vi "LurchTowardsPoint.vi"(2 "Turning Radius (m) \n(Goes into Dillons' Movement Control)":dbl=1.75, 3 "Robot Speed":dbl(slide)=1.0 scale=0.0..1.0, 4 "Reached Next Path Point Threshold Distance (m)":dbl(knob)=0.4965904536247452 scale=0.0..1.0, 5 "Dest. Point":cluster{"x":dbl, "y":dbl}, 7 "Curr Localization Status":T1) -> (0 "Within Tolerance of Dest":bool, 1 "Distance to Dest Point (m)":dbl)   [LabVIEW 2015, in "Navigation2017.lvlib"]
doc: "Tries to move the robot one \"jump\" forward towards (or even to) a given point. Uses a time measured in the testing arena to determine a minimum time to move robot forward, erring on the side of undershooting the target point on BP-1. Likely will not exactly reach the final point, as dead reckoning is used to move bot until it stops and checks its location again."
uses:
  Navigation2017.lvlib
  LocalizationStatus.ctl
  Navigation2017-util.lvlib
  MovementControl2017.lvlib
  Navigation2017-SubVIs.lvlib
panel:
  in  "Time to move 1m (TODO: consider speed?)":u32=1
  # "INTERNAL VALUE\nTO VI:"
  # "INPUTS"
  # "OUTPUTS:"
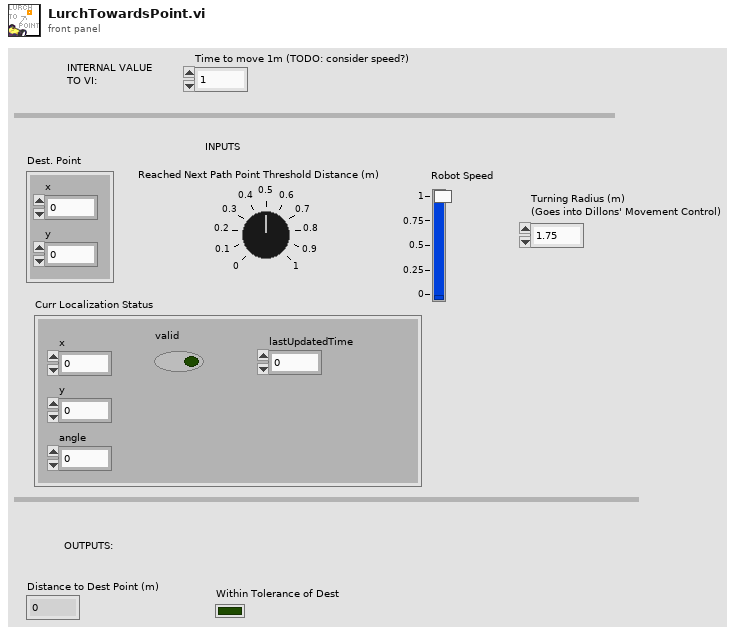
[diagram p1: front panel]
types:
  T1 = typedef "LocalizationStatus.ctl" = cluster{"x":dbl, "y":dbl, "angle":dbl, "valid":bool, "lastUpdatedTime":dbl}
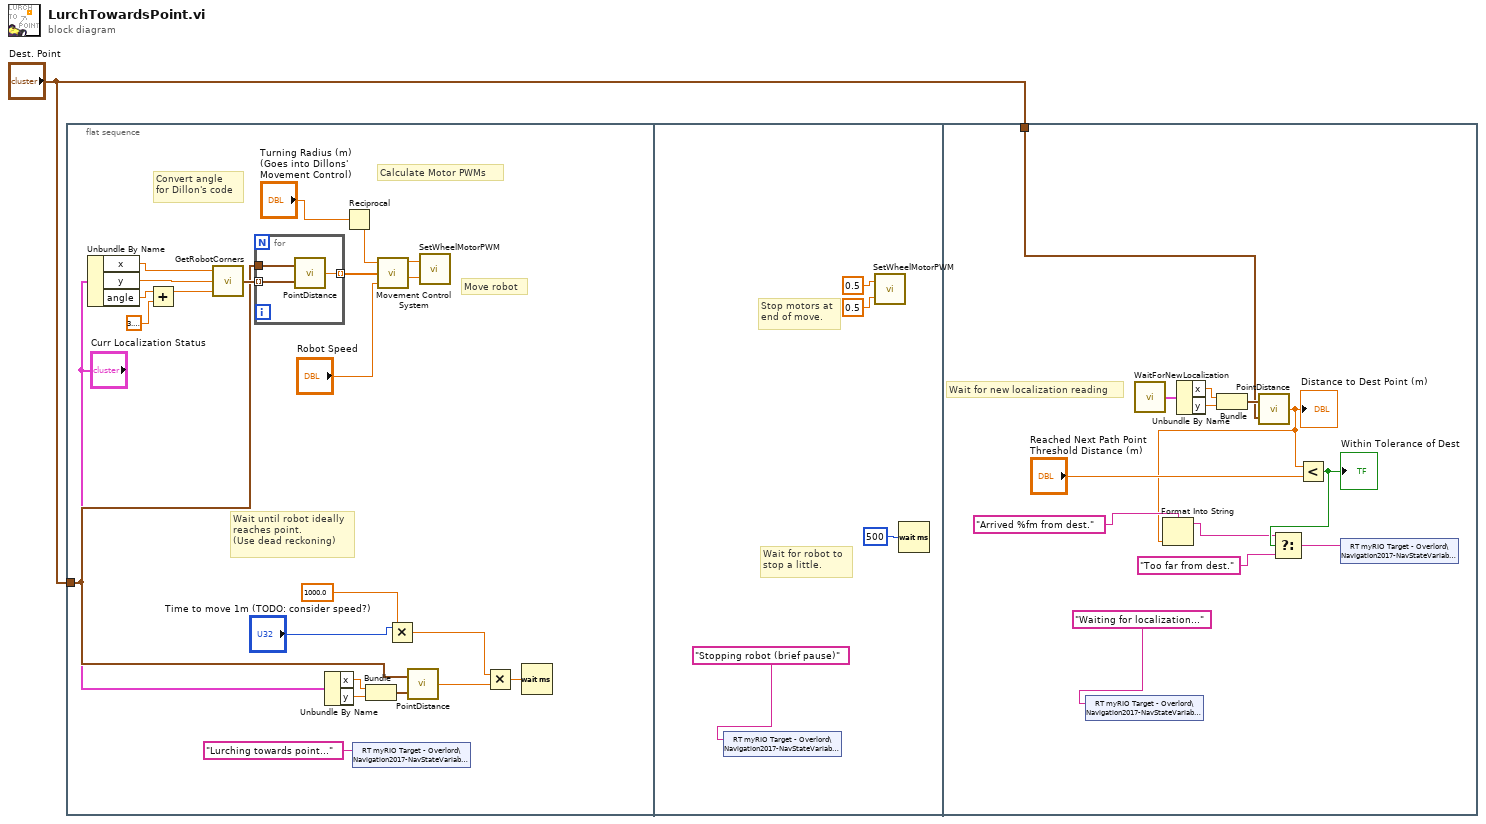
[diagram p0: block diagram]
diagram:
  n1 = flat-sequence {
    tunnel: "Dest. Point" -> [w12]
    tunnel: "Dest. Point" -> [w39]
    frame #0 {
      # "Convert angle\nfor Dillon's code"
      # "Move robot"
      # "Wait until robot ideally\nreaches point.\n(Use dead reckoning)"
      # "Calculate Motor PWMs"
      n2 = Unbundle By Name("Curr Localization Status") -> ("x"=w22:dbl, "y"=w21:dbl, "angle"=w4:dbl)
      n3 = Add(x=w4, y=3.141592653589793) -> (x+y=w3:dbl)
      n4 = call "GetRobotCorners.vi"("botAngle (rad)"=w3, "botY (m)"=w21, "botX (m)"=w22) -> ("Corner Points (m)"=w24:cluster{dbl, dbl}[])
      n5 = for {
        tunnel: w24 -> [w26] mode=indexing
        tunnel: [w25] -> w23 mode=indexing
        tunnel: w12 -> [w27]
        n6 = call "PointDistance.vi"("Point 2"=w26, "Point 1"=w27) -> ("Distance"=w25:dbl)
      }
      n7 = Unbundle By Name("Curr Localization Status") -> ("x"=w15:dbl, "y"=w14:dbl)
      n8 = Reciprocal(x="Turning Radius (m) \n(Goes into Dillons' Movement Control)") -> (1/x=w9:dbl)
      n9 = shared-variable "RT myRIO Target - Overlord\\Navigation2017-NavStateVariables.lvlib\\CurrNavStage"("Lurching towards point..." ("CurrNavStage")) -> ()  [unwired: 1 in, 1 out]
      n10 = Bundle("x"=w15, "y"=w14) -> (w13:cluster{"x":dbl, "y":dbl})  [unwired: 1 in]
      n11 = call "Movement Control System.vi"("Turning Radius"=w9, "Corner Distances"=w23, "Speed"="Robot Speed") -> ("Left Side PWM"=w20:dbl, "Right Side PWM"=w19:dbl)  [unwired: 4 out]
      n12 = Multiply(x="Time to move 1m (TODO: consider speed?)", y=1000.0) -> (x*y=w6:dbl)
      n13 = call "PointDistance.vi"("Point 2"=w13, "Point 1"=w12) -> ("Distance"=w17:dbl)
      n14 = call "SetWheelMotorPWM.vi"("Right Motor PWM"=w19, "Left Motor PWM"=w20) -> ()
      n15 = Multiply(x=w6, y=w17) -> (x*y=w16:dbl)
      n16 = Wait (ms)(milliseconds to wait=w16) -> ()  [unwired: 1 out]
    }
    frame #1 {
      # "Wait for robot to\nstop a little."
      # "Stop motors at\nend of move."
      n17 = shared-variable "RT myRIO Target - Overlord\\Navigation2017-NavStateVariables.lvlib\\CurrNavStage"("Stopping robot (brief pause)" ("CurrNavStage")) -> ()  [unwired: 1 in, 1 out]
      n18 = call "SetWheelMotorPWM.vi"("Right Motor PWM"=0.5 ("Right Motor Speed"), "Left Motor PWM"=0.5 ("Left Motor Speed")) -> ()
      n19 = Wait (ms)(milliseconds to wait=u32 500) -> ()  [unwired: 1 out]
    }
    frame #2 {
      # "Wait for new localization reading"
      n20 = shared-variable "RT myRIO Target - Overlord\\Navigation2017-NavStateVariables.lvlib\\CurrNavStage"("Waiting for localization..." ("CurrNavStage")) -> ()  [unwired: 1 in, 1 out]
      n21 = call "WaitForNewLocalization.vi"() -> ("Localization Status"=w44:T1)
      n22 = Unbundle By Name(w44) -> ("x"=w43:dbl, "y"=w42:dbl)
      n23 = Bundle("x"=w43, "y"=w42) -> (w41:cluster{"x":dbl, "y":dbl})  [unwired: 1 in]
      n24 = call "PointDistance.vi"("Point 2"=w39, "Point 1"=w41) -> ("Distance"=w32:dbl)
      "Distance to Dest Point (m)" <- w32
      n25 = Format Into String(format string="Arrived %fm from dest." ("string"), w32) -> (resulting string=w34:string)  [unwired: 2 in, 1 out]
      n26 = Less?(x=w32, y="Reached Next Path Point Threshold Distance (m)") -> (x < y?=w36:bool)
      "Within Tolerance of Dest" <- w36
      n27 = Select(t=w34, s=w36, f="Too far from dest.") -> (s? t:f=w37:string)
      n28 = shared-variable "RT myRIO Target - Overlord\\Navigation2017-NavStateVariables.lvlib\\CurrNavStage"(w37) -> ()  [unwired: 1 in, 1 out]
    }
  }
